vi "Save 8-Contact Sample test results to Disk.vi"(0 "Save To Path":path, 1 "Sample Name":string, 2 "User Name":string, 3 "Test Date":string, 5 "Test Settings":T3={"Current Level"=0.0, "Compliance Level"=0.0, "Soak Time"=0.0, "NPLC Voltmeter"=1.0, "Count Voltmeter"=1, "NPLC Ammeter"=1.0, "Count Ammeter"=1, "Sample Resistivity"=enum."Low", "Sample Thickness"=0.0, "Magnetic Flux"=0.0, "Units"=enum."T", "Sample Dimensions x"=0.0, "Sample Dimensions y"=0.0, "Sample Dimensions D1"=0.0, "Sample Dimensions D2"=0.0, "Sample Width Ws"=0.0, "Slot Number of 3765 card"=1} {"Slot Number of 3765 card" min=1 max=6; "NPLC Ammeter" min=0.01 max=10.0; "NPLC Voltmeter" min=0.01 max=10.0 format="%^#_6g"; "Count Ammeter" min=1 max=1024; "Count Voltmeter" min=1 max=1024; "Soak Time" format="%^#_6g"; "Compliance Level" format="%^#_6g"; "Current Level" format="%^#_6e"}, 11 "error in (no error)":errorcluster, 12 "8-Contact Sample Resitivity Measurements":cluster{"V1":dbl, "V2":dbl, "V3":dbl, "V4":dbl}, 13 "8-Contact Sample Hall Voltage Measurements":cluster{"V1":dbl, "V2":dbl, "V3":dbl, "V4":dbl}, 14 "8-Contact Sample Results":T1) -> (15 "error out":errorcluster)   [LabVIEW 2016]
uses:
  Hall Effect Library/Public/Controls/Resisitivity.ctl
  Hall Effect Library/Hall Effect Library.lvlib
panel:
  # "Hall Coefficient"
  # "Hall Mobility"
  # "Resistivity"
  # "Ohm cm"
  # "PAvg"
  # "uH"
  # "RH"
  # "cm^3/C"
  # "cm^2/V s"
  # "Ohm cm"
  # "PA"
  # "PB"
  # "Ohm cm"
  # "V1"
  # "Magnet"
  # "V2"
  # "Pos"
  # "Volts"
  # "Neg"
  # "Polarity"
  # "V4"
  # "V3"
  # "V1"
  # "Currents"
  # "V2"
  # "Pos"
  # "Volts"
  # "Neg"
  # "Direction"
  # "V4"
  # "V3"
  # "NPLC"
  # "A"
  # "V"
  # "s"
  # "Measure Count"
  # "cm"
  # "cm"
  # "cm"
  # "cm"
  # "cm"
  # "cm"
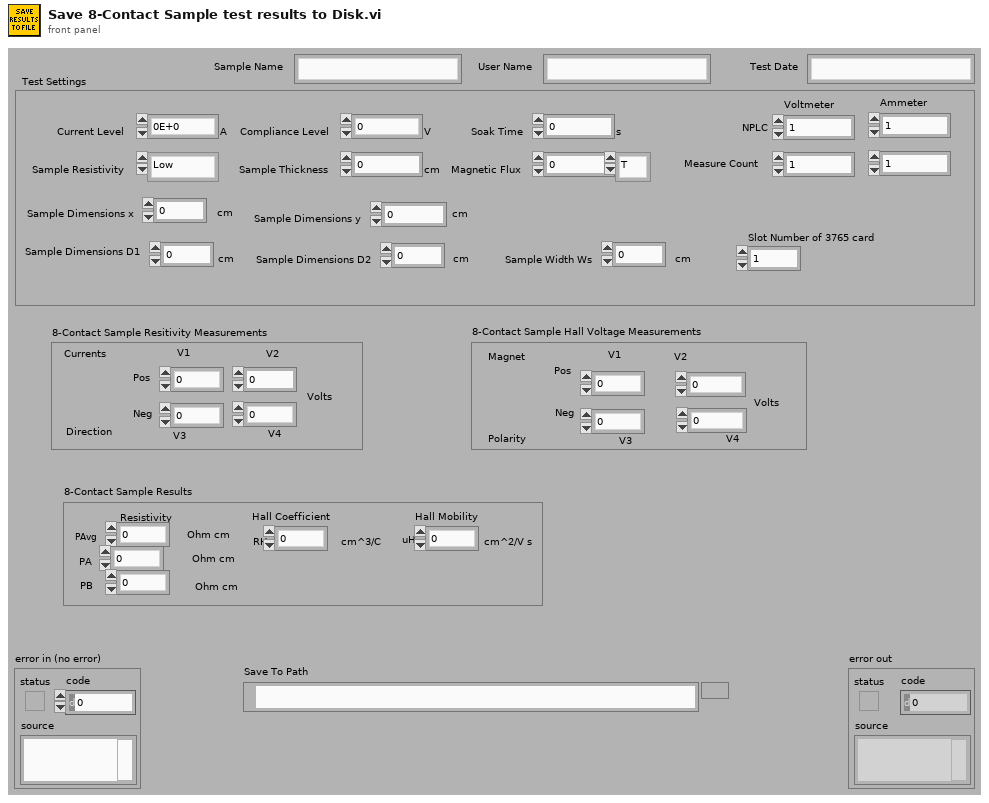
[diagram p1: front panel]
types:
  T1 = cluster{"Pavg":dbl, "PA":dbl, "PB":dbl, "RAVG":dbl, "uH":dbl}
  T2 = typedef "Hall Effect Library.lvlib/Resisitivity.ctl" = enum16{"Low", "High"}
  T3 = cluster{"Current Level":dbl, "Compliance Level":dbl, "Soak Time":dbl, "NPLC Voltmeter":dbl, "Count Voltmeter":i32, "NPLC Ammeter":dbl, "Count Ammeter":i32, "Sample Resistivity":T2, "Sample Thickness":dbl, "Magnetic Flux":dbl, "Units":enum16{"Gs", "T"}, "Sample Dimensions x":dbl, "Sample Dimensions y":dbl, "Sample Dimensions D1":dbl, "Sample Dimensions D2":dbl, "Sample Width Ws":dbl, "Slot Number of 3765 card":u16}
  T4 = enum16{"open", "replace", "create", "open or create", "replace or create", "replace or create with confirmation"}
  T5 = cluster{"8-Contact Sample Resistivity Currents[0]":dbl, "8-Contact Sample Resistivity Currents[1]":dbl, "8-Contact Sample Resistivity Currents[2]":dbl, "8-Contact Sample Resistivity Currents[3]":dbl}
  T6 = cluster{"8-Contact Sample Hall Currents[0]":dbl, "8-Contact Sample Hall Currents[1]":dbl, "8-Contact Sample Hall Currents[2]":dbl, "8-Contact Sample Hall Currents[3]":dbl, "8-Contact Sample Hall Currents[4]":dbl, "8-Contact Sample Hall Currents[5]":dbl, "8-Contact Sample Hall Currents[6]":dbl, "8-Contact Sample Hall Currents[7]":dbl, "8-Contact Sample Hall Currents[8]":dbl}
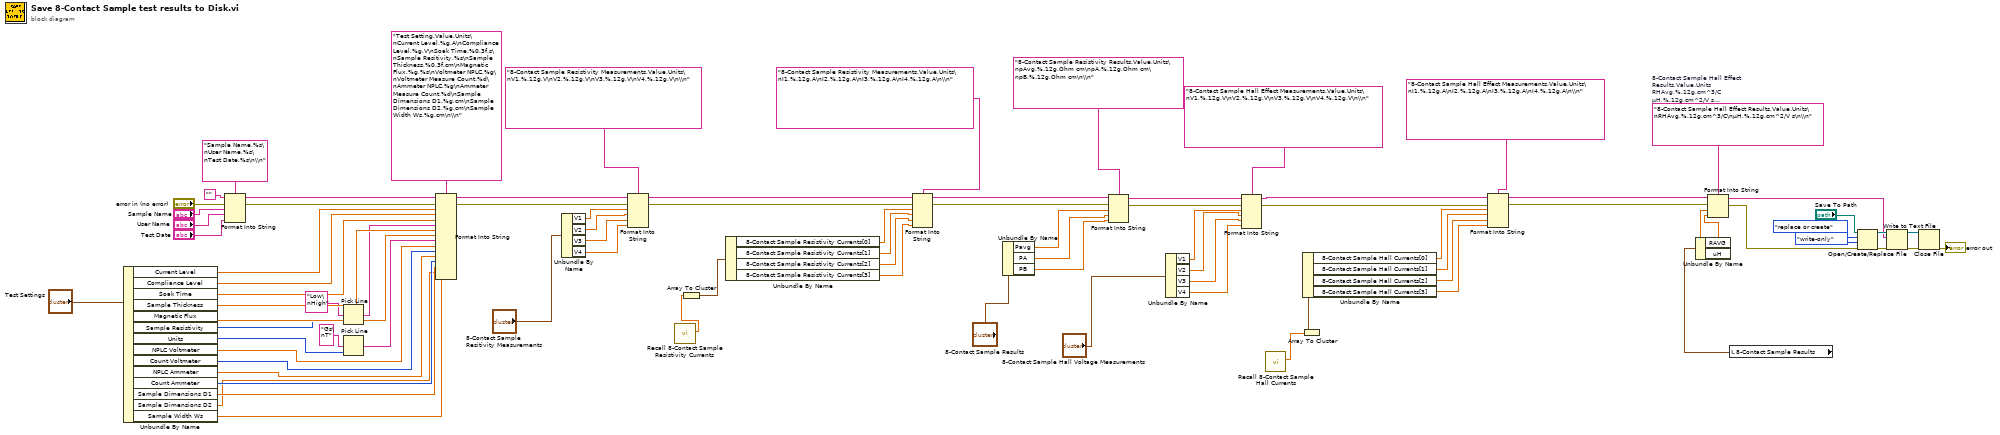
[diagram p0: block diagram]
diagram:
  w58 = "8-Contact Sample Hall Effect Results,Value,Units\nRHAvg,%.12g,cm^3/C\nµH,%.12g,cm^2/V s\n\\n"  # 8-Contact Sample Hall Effect Results,Value,Units RHAvg,%.12g,cm^3/C µH,%.12g,cm^2/V s \n
  n1 = Unbundle By Name("Test Settings") -> ("Current Level"=w78:dbl, "Compliance Level"=w77:dbl, "Soak Time"=w76:dbl, "Sample Thickness"=w75:dbl, "Magnetic Flux"=w74:dbl, "Sample Resistivity"=w70:T2, "Units"=w71:enum16{"Gs", "T"}, "NPLC Voltmeter"=w46:dbl, "Count Voltmeter"=w45:i32, "NPLC Ammeter"=w44:dbl, "Count Ammeter"=w43:i32, "Sample Dimensions D1"=w42:dbl, "Sample Dimensions D2"=w41:dbl, "Sample Width Ws"=w40:dbl)
  n2 = Format Into String(format string="Sample Name,%s\nUser Name,%s\nTest Date,%s\n\\n", initial string="", error in="error in (no error)", "Sample Name", "User Name", "Test Date") -> (resulting string=w66:string, error out=w67:errorcluster)
  n3 = Pick Line(multi-line string="Low\nHigh", line index=w70) -> (output string=w69:string)  [unwired: 1 out]
  n4 = Pick Line(multi-line string="Gs\nT", line index=w71) -> (output string=w68:string)  [unwired: 1 out]
  n5 = Format Into String(format string="Test Setting,Value,Units\nCurrent Level,%g,A\nCompliance Level,%g,V\nSoak Time,%0.3f,s\nSample Resitivity,%s\nSample Thickness,%0.3f,cm\nMagnetic Flux,%g,%s\nVoltmeter NPLC,%g\nVoltmeter Measure Count,%d\nAmmeter NPLC,%g\nAmmeter Measure Count,%d\nSample Dimensions D1,%g,cm\nSample Dimensions D2,%g,cm\nSample Width Ws,%g,cm\n\\n", initial string=w66, error in=w67, w78, w77, w76, w69, w75, w74, w68, w46, w45, w44, w43, w42, w41, w40) -> (resulting string=w64:string, error out=w63:errorcluster)
  n6 = Unbundle By Name("8-Contact Sample Resitivity Measurements") -> ("V1"=w38:dbl, "V2"=w37:dbl, "V3"=w36:dbl, "V4"=w35:dbl)
  n7 = Format Into String(format string="8-Contact Sample Resistivity Measurements,Value,Units\nV1,%.12g,V\nV2,%.12g,V\nV3,%.12g,V\nV4,%.12g,V\n\\n", initial string=w64, error in=w63, w38, w37, w36, w35) -> (resulting string=w20:string, error out=w19:errorcluster)
  n8 = call "Recall 8-Contact Sample Resistivity Currents.vi"() -> ("8-Contact Sample Resistivity Currents"=w22:dbl[])  [unwired: 11 in]
  n9 = Array To Cluster(array=w22) -> (cluster=w21:T5)
  n10 = Unbundle By Name(w21) -> ("8-Contact Sample Resistivity Currents[0]"=w18:dbl, "8-Contact Sample Resistivity Currents[1]"=w17:dbl, "8-Contact Sample Resistivity Currents[2]"=w16:dbl, "8-Contact Sample Resistivity Currents[3]"=w15:dbl)
  n11 = Format Into String(format string="8-Contact Sample Resistivity Measurements,Value,Units\nI1,%.12g,A\nI2,%.12g,A\nI3,%.12g,A\nI4,%.12g,A\n\\n", initial string=w20, error in=w19, w18, w17, w16, w15) -> (resulting string=w14:string, error out=w13:errorcluster)
  n12 = Unbundle By Name("8-Contact Sample Results") -> ("Pavg"=w33:dbl, "PA"=w32:dbl, "PB"=w31:dbl)
  n13 = Format Into String(format string="8-Contact Sample Resistivity Results,Value,Units\npAvg,%.12g,Ohm cm\npA,%.12g,Ohm cm\npB,%.12g,Ohm cm\n\\n", initial string=w14, error in=w13, w33, w32, w31) -> (resulting string=w60:string, error out=w59:errorcluster)
  n14 = Unbundle By Name("8-Contact Sample Hall Voltage Measurements") -> ("V1"=w29:dbl, "V2"=w28:dbl, "V3"=w27:dbl, "V4"=w26:dbl)
  n15 = Format Into String(format string="8-Contact Sample Hall Effect Measurements,Value,Units\nV1,%.12g,V\nV2,%.12g,V\nV3,%.12g,V\nV4,%.12g,V\n\\n", initial string=w60, error in=w59, w29, w28, w27, w26) -> (resulting string=w5:string, error out=w4:errorcluster)
  n16 = call "Recall 8-Contact Sample Hall Currents.vi"() -> ("8-Contact Sample Hall Currents"=w11:dbl[])  [unwired: 11 in]
  n17 = Array To Cluster(array=w11) -> (cluster=w10:T6)
  n18 = Unbundle By Name(w10) -> ("8-Contact Sample Hall Currents[0]"=w9:dbl, "8-Contact Sample Hall Currents[1]"=w8:dbl, "8-Contact Sample Hall Currents[2]"=w7:dbl, "8-Contact Sample Hall Currents[3]"=w6:dbl)
  n19 = Format Into String(format string="8-Contact Sample Hall Effect Measurements,Value,Units\nI1,%.12g,A\nI2,%.12g,A\nI3,%.12g,A\nI4,%.12g,A\n\\n", initial string=w5, error in=w4, w9, w8, w7, w6) -> (resulting string=w3:string, error out=w2:errorcluster)
  n20 = local read "8-Contact Sample Results"() -> (w25:T1)
  n21 = Unbundle By Name(w25) -> ("RAVG"=w24:dbl, "uH"=w23:dbl)
  n22 = Format Into String(format string=w58, initial string=w3, error in=w2, w24, w23) -> (resulting string=w49:string, error out=w50:errorcluster)
  n23 = Open/Create/Replace File(file path (use dialog)="Save To Path", error in=w50, operation (0:open)=T4."replace or create", access (0:read/write)=enum16{"read/write", "read-only", "write-only"}."write-only") -> (refnum out=w54:refnum<file>, error out=w53:errorcluster)  [unwired: 3 out]
  n24 = Write to Text File(file (use dialog)=w54, text=w49, error in=w53) -> (refnum out=w51:refnum<file>, error out=w52:errorcluster)  [unwired: 2 out]
  n25 = Close File(refnum=w51, error in=w52) -> (error out=→"error out":errorcluster)  [unwired: 1 out]
